vi "aaaaa.vi"() -> ()   [LabVIEW 2024]
panel:
  out "OutputValue":string
  out "appended path":path
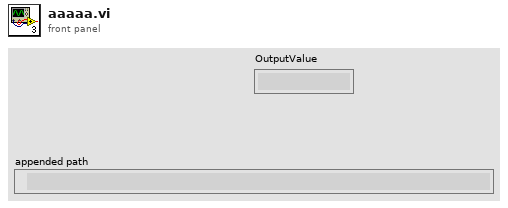
[diagram p1: front panel]
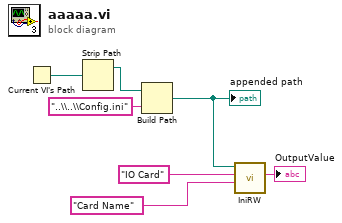
[diagram p0: block diagram]
diagram:
  n1 = Current VI's Path() -> (path=w7:path)
  n2 = Strip Path(path=w7) -> (stripped path=w6:path)  [unwired: 1 out]
  n3 = Build Path(base path=w6, name or relative path="..\\..\\Config.ini") -> (appended path=w4:path)
  "appended path" <- w4
  n4 = call "IniRW.vi"("Key"="Card Name", "Section"="IO Card", "IniFilePath"=w4) -> ("OutputValue"=→"OutputValue":string)  [unwired: 6 in, 2 out]
